vi "Read TemperatureSettling.vi"(11 "TestMonitor in":refnum<class "TestMonitor.lvclass">) -> (2 "TemperatureSettling":T1={"Temperature Measured"=275.15, "TemperatureSettledIsTrue"=FALSE, "Required"={"Sample Size Rqd"=0, "StDev"=275.15}, "Measured"={"StDev Msd"=275.15, "Sample Size Msd"=0}} {"Measured"."StDev Msd" min=271.15 max=275.15 format="%.4f"; "Measured"."Sample Size Msd" min=1; "Required"."Sample Size Rqd" min=1; "Required"."StDev" min=271.15 max=275.15 format="%.4f"; "Temperature Measured" min=271.15 max=275.15 format="%.1f"}, 3 "TestMonitor out":refnum<class "TestMonitor.lvclass">)   [LabVIEW 2013, in "TestMonitor.lvclass"]
uses:
  TestMonitor.lvclass
  Typedefs/TemperatureSettling.ctl
  TestMonitor.lvclass/TestMonitor.ctl
  Typedefs/AITDTTypedefs.lvlib
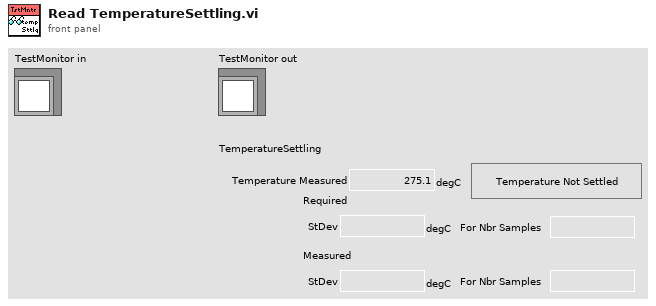
[diagram p1: front panel]
types:
  T1 = typedef "AITDTTypedefs.lvlib/TemperatureSettling.ctl" = cluster{"Temperature Measured":dbl[unit], "TemperatureSettledIsTrue":bool, "Required":cluster{"Sample Size Rqd":u16, "StDev":dbl[unit]}, "Measured":cluster{"StDev Msd":dbl[unit], "Sample Size Msd":u16}}
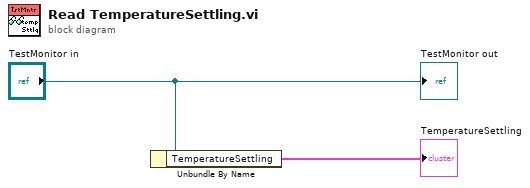
[diagram p0: block diagram]
diagram:
  n1 = Unbundle By Name("TestMonitor in") -> ("TemperatureSettling"=→"TemperatureSettling":T1)
  "TestMonitor out" <- "TestMonitor in"
